vi "NumericArraytoIgorWave.vi"(8 "error in (no error)":errorcluster, 10 "Wave":dbl[](array[numeric]), 11 "Name":string) -> (0 "error out":errorcluster, 3 "Igor Wave":string)   [LabVIEW 2016]
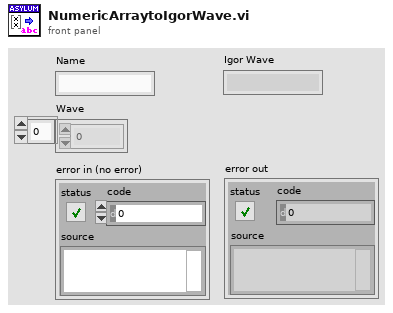
[diagram p1: front panel]
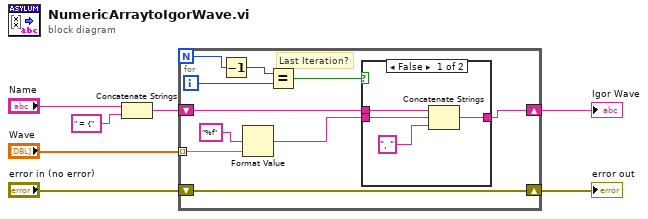
[diagram p0: block diagram]
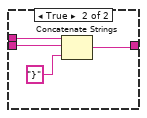
[diagram p2: hidden frame]
diagram:
  n1 = Concatenate Strings("Name", " = {" ("string")) -> (w7:string)
  n2 = for {
    N -> [w15]
    tunnel: "Wave" -> [w11] mode=indexing
    shift-right: [w16] -> w1
    shift-left: w7 -> [w17]
    shift-right: [w8] -> w4
    shift-left: "error in (no error)" -> [w8]
    i -> [w13]
    # "Last Iteration?"
    n3 = Decrement(x=w15) -> (x-1=w14:i32)
    n4 = Format Value(format string="%f", value (0)=w11) -> (output string=w10:string)  [unwired: 1 in]
    n5 = Equal?(x=w14, y=w13) -> (x = y?=w12:bool)
    n6 = case shown="False" w12 {
      tunnel: w17 -> [w21 w25]
      tunnel: w10 -> [w20 w24]
      tunnel: [w18 w22] -> w16
      frame False {
        n7 = Concatenate Strings(w21, w20, ", " ("string")) -> (w18:string)
      }
      frame True {
        n8 = Concatenate Strings(w25, w24, "}") -> (w22:string)
      }
    }
  }
  "error out" <- w4
  "Igor Wave" <- w1
